vi "GenerateCode.vi"(0 "XRef":T11, 1 "Terms":T8, 2 "Diagram":T7, 3 "State In":T1) -> (14 "Generated Code?":T6, 15 "Reply":T4, 16 "Fatal Error Out":T3, 17 "State Out":T1)   [LabVIEW 2015, in "LVJSON.lvlib" / "Set Object Parameters.xnode"]
uses:
  Set Object Parameters.xnode
  <vilib>/XNodeSupport/XNodeXNodeRef.ctl
  <vilib>/XNodeSupport/XNodeTermIDPairs.ctl
  <vilib>/XNodeSupport/XNodeTermIDPair.ctl
  <vilib>/XNodeSupport/XNodeTermRef.ctl
  <vilib>/XNodeSupport/XNodeString.ctl
  <vilib>/XNodeSupport/XNodeTopLevelDiagramRef.ctl
  State.ctl
  Get Object Parameters/Parameter.ctl
  <vilib>/XNodeSupport/XNodeBool.ctl
  <vilib>/XNodeSupport/XNodeStringArray.ctl
  <vilib>/XNodeSupport/XNodeErrorCluster.ctl
  <vilib>/Utility/miscctls.llb/LVPointTypeDef.ctl
  Insert Key Value Pair.vi
  <vilib>/XNodeSupport/NI_XNodeSupport.lvlib
  JSON Object.lvclass
  Shared/Shared.lvlib
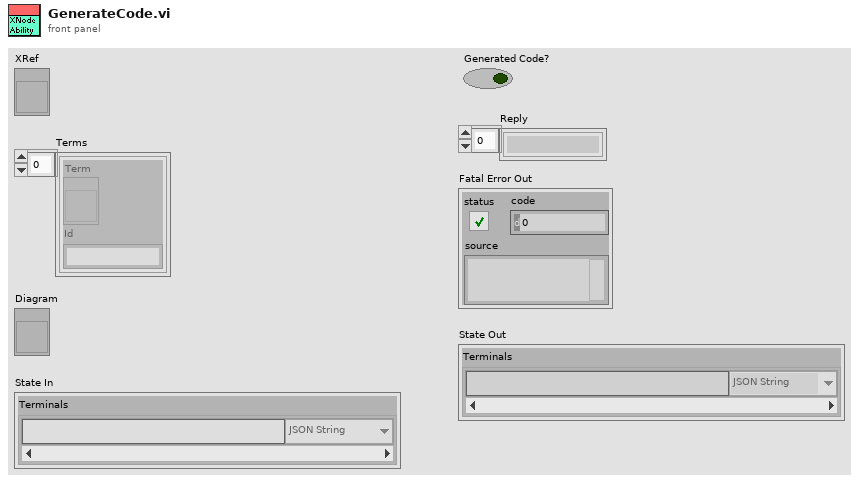
[diagram p1: front panel]
types:
  T1 = typedef "LVJSON.lvlib/Set Object Parameters.xnode/State.ctl" = cluster{"Terminals":T2[]}
  T2 = typedef "LVJSON.lvlib/Shared.lvlib/Parameter.ctl" = cluster{"Parameter Name":string, "JSON Type":enum16{"JSON String", "JSON Numeric", "JSON Boolean", "JSON", "JSON Object", "JSON Array", "String Value", "Numeric Value", "Boolean Value"}}
  T3 = typedef "NI_XNodeSupport.lvlib/XNodeErrorCluster.ctl" = errorcluster
  T4 = typedef "NI_XNodeSupport.lvlib/XNodeStringArray.ctl" = T5[]
  T5 = typedef "NI_XNodeSupport.lvlib/XNodeString.ctl" = string
  T6 = typedef "NI_XNodeSupport.lvlib/XNodeBool.ctl" = bool
  T7 = typedef "NI_XNodeSupport.lvlib/XNodeTopLevelDiagramRef.ctl" = refnum<vi>
  T8 = typedef "NI_XNodeSupport.lvlib/XNodeTermIDPairs.ctl" = T9[]
  T9 = typedef "NI_XNodeSupport.lvlib/XNodeTermIDPair.ctl" = cluster{"Term":T10, "Id":T5}
  T10 = typedef "NI_XNodeSupport.lvlib/XNodeTermRef.ctl" = refnum<vi>
  T11 = typedef "NI_XNodeSupport.lvlib/XNodeXNodeRef.ctl" = refnum<vi>
  T12 = typedef "LVPointTypeDef.ctl" = cluster{"Horizontal":i16, "Vertical":i16}
  T13 = enum16{"JSON String", "JSON Numeric", "JSON Boolean", "JSON", "JSON Object", "JSON Array", "String Value", "Numeric Value", "Boolean Value"}
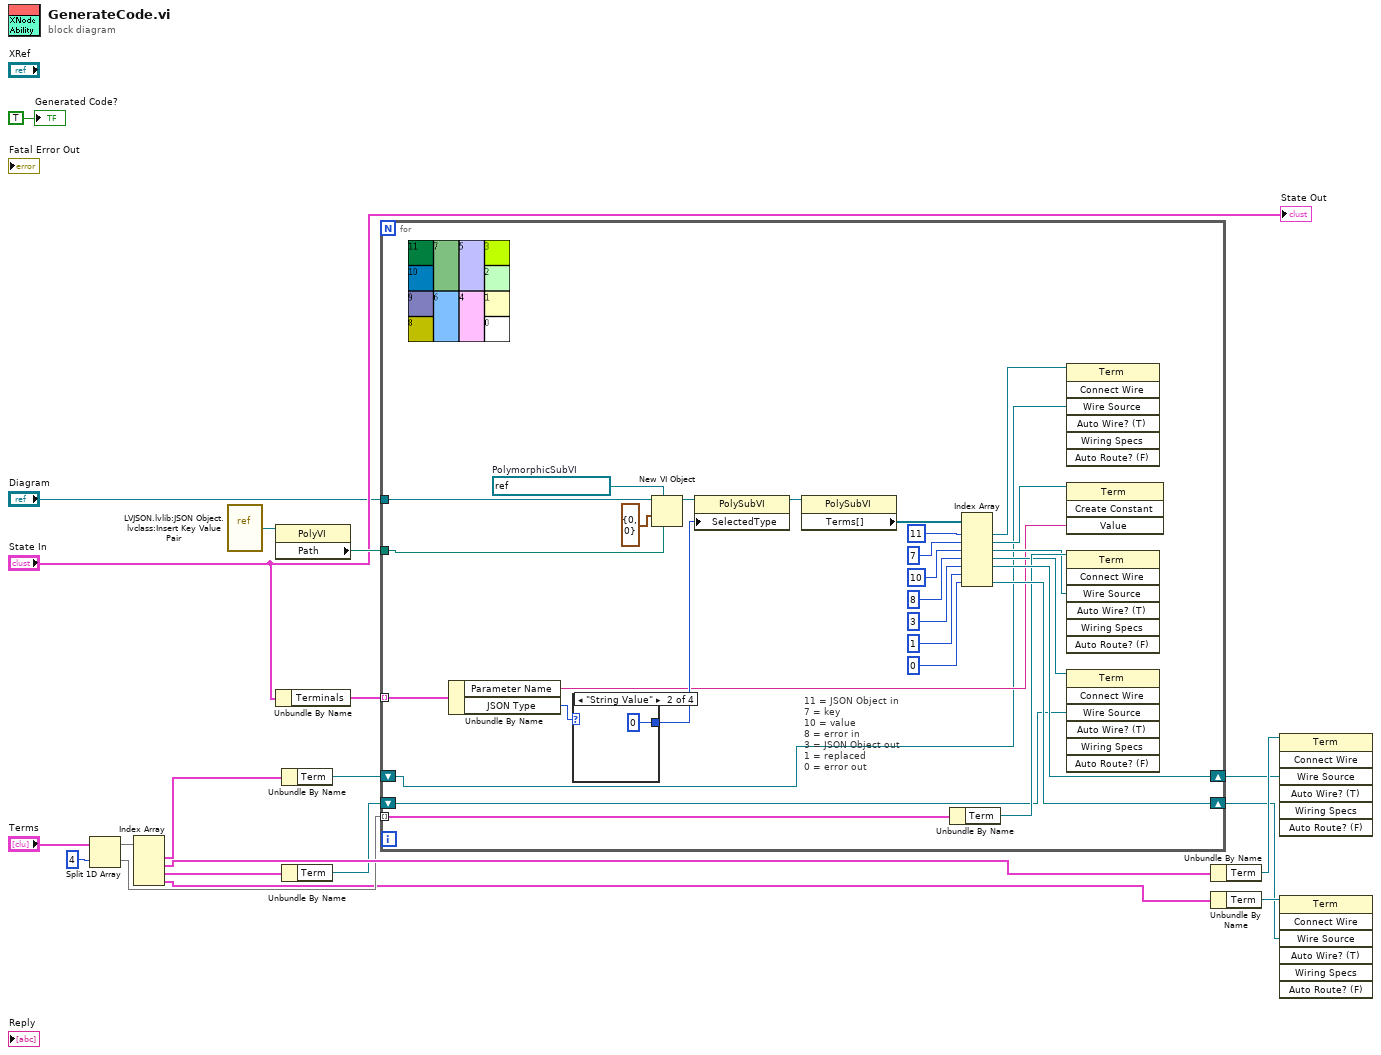
[diagram p0: block diagram]
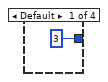
[diagram p2: hidden frame]
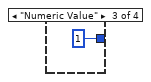
[diagram p3: hidden frame]
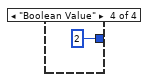
[diagram p4: hidden frame]
diagram:
  n1 = Split 1D Array(array="Terms", index=4) -> (first subarray=w16:T8, second subarray=w14:T8)
  n2 = Index Array(array=w16) -> (element #1=w15:T9, element #2=w19:T9, element #3=w9:T9, element #4=w6:T9)  [unwired: 4 in]
  n3 = vi-ref "LVJSON.lvlib:JSON Object.lvclass:Insert Key Value Pair.vi"() -> (w12:refnum<vi>)
  n4 = property class="PolyVI"(reference=w12) -> ("Path"=w13:path)  [unwired: 1 in, 2 out]
  n5 = Unbundle By Name("State In") -> ("Terminals"=w7:T2[])
  n6 = Unbundle By Name(w15) -> ("Term"=w11:T10)
  n7 = Unbundle By Name(w9) -> ("Term"=w5:T10)
  n8 = for {
    tunnel: w14 -> [w48] mode=indexing
    tunnel: "Diagram" -> [w47]
    tunnel: w13 -> [w44]
    tunnel: w7 -> [w41] mode=indexing
    shift-right: [w30] -> w3
    shift-left: w11 -> [w21]
    shift-right: [w29] -> w1
    shift-left: w5 -> [w25]
    w46 = refnum<vi> refnum  # PolymorphicSubVI
    # "11 = JSON Object in\n7 = key\n10 = value\n8 = error in\n3 = JSON Object out\n1 = replaced\n0 = error out"
    n9 = Unbundle By Name(w41) -> ("Parameter Name"=w23:string, "JSON Type"=w40:T13)
    n10 = case shown="\"String Value\"" w40 {
      tunnel: [3 0 1 2] -> w39
      frame Default {
      }
      frame "String Value" {
      }
      frame "Numeric Value" {
      }
      frame "Boolean Value" {
      }
    }
    n11 = New VI Object(vi object class=w46, owner refnum=w47, position/next to=T12 {"Horizontal"=0, "Vertical"=0} ("location"), 6:w44) -> (object refnum=w38:refnum<vi>)  [unwired: 4 in, 1 out]
    n12 = property class="PolySubVI"(reference=w38, "SelectedType"=w39) -> (reference out=w37:refnum<vi>)  [unwired: 1 in, 1 out]
    n13 = property class="PolySubVI"(reference=w37) -> ("Terms[]"=w43:refnum<vi>[])  [unwired: 1 in, 2 out]
    n14 = Unbundle By Name(w48) -> ("Term"=w28:T10)
    n15 = Index Array(array=w43, index #1=11 ("index"), index #2=7 ("index"), index #3=10 ("index"), index #4=8 ("index"), index #5=3 ("index"), index #6=1 ("index"), index #7=0 ("index")) -> (element #1=w22:refnum<vi>, element #2=w24:refnum<vi>, element #3=w27:refnum<vi>, element #4=w26:refnum<vi>, element #5=w30:refnum<vi>, element #7=w29:refnum<vi>)  [unwired: 1 out]
    n16 = invoke class="Term" method="Connect Wire"(reference=w22, "Wire Source"=w21) -> ()  [unwired: 5 in, 7 out]
    n17 = invoke class="Term" method="Create Constant"(reference=w24, "Value"=w23) -> ()  [unwired: 2 in, 4 out]
    n18 = invoke class="Term" method="Connect Wire"(reference=w28, "Wire Source"=w27) -> ()  [unwired: 5 in, 7 out]
    n19 = invoke class="Term" method="Connect Wire"(reference=w26, "Wire Source"=w25) -> ()  [unwired: 5 in, 7 out]
  }
  n20 = Unbundle By Name(w19) -> ("Term"=w4:T10)
  n21 = Unbundle By Name(w6) -> ("Term"=w2:T10)
  n22 = invoke class="Term" method="Connect Wire"(reference=w4, "Wire Source"=w3) -> ()  [unwired: 5 in, 7 out]
  n23 = invoke class="Term" method="Connect Wire"(reference=w2, "Wire Source"=w1) -> ()  [unwired: 5 in, 7 out]
  "Generated Code?" <- T6 TRUE ("Generated Code?")
  "State Out" <- "State In"
